vi "Save Properties as XML.vi"(8 "error in":errorcluster, 9 "Methods[]":T1(array[cluster]), 10 "Properties[]":T2(array[cluster]), 11 "Classes":T3(array[cluster])) -> (0 "error out":errorcluster)   [LabVIEW 2023]
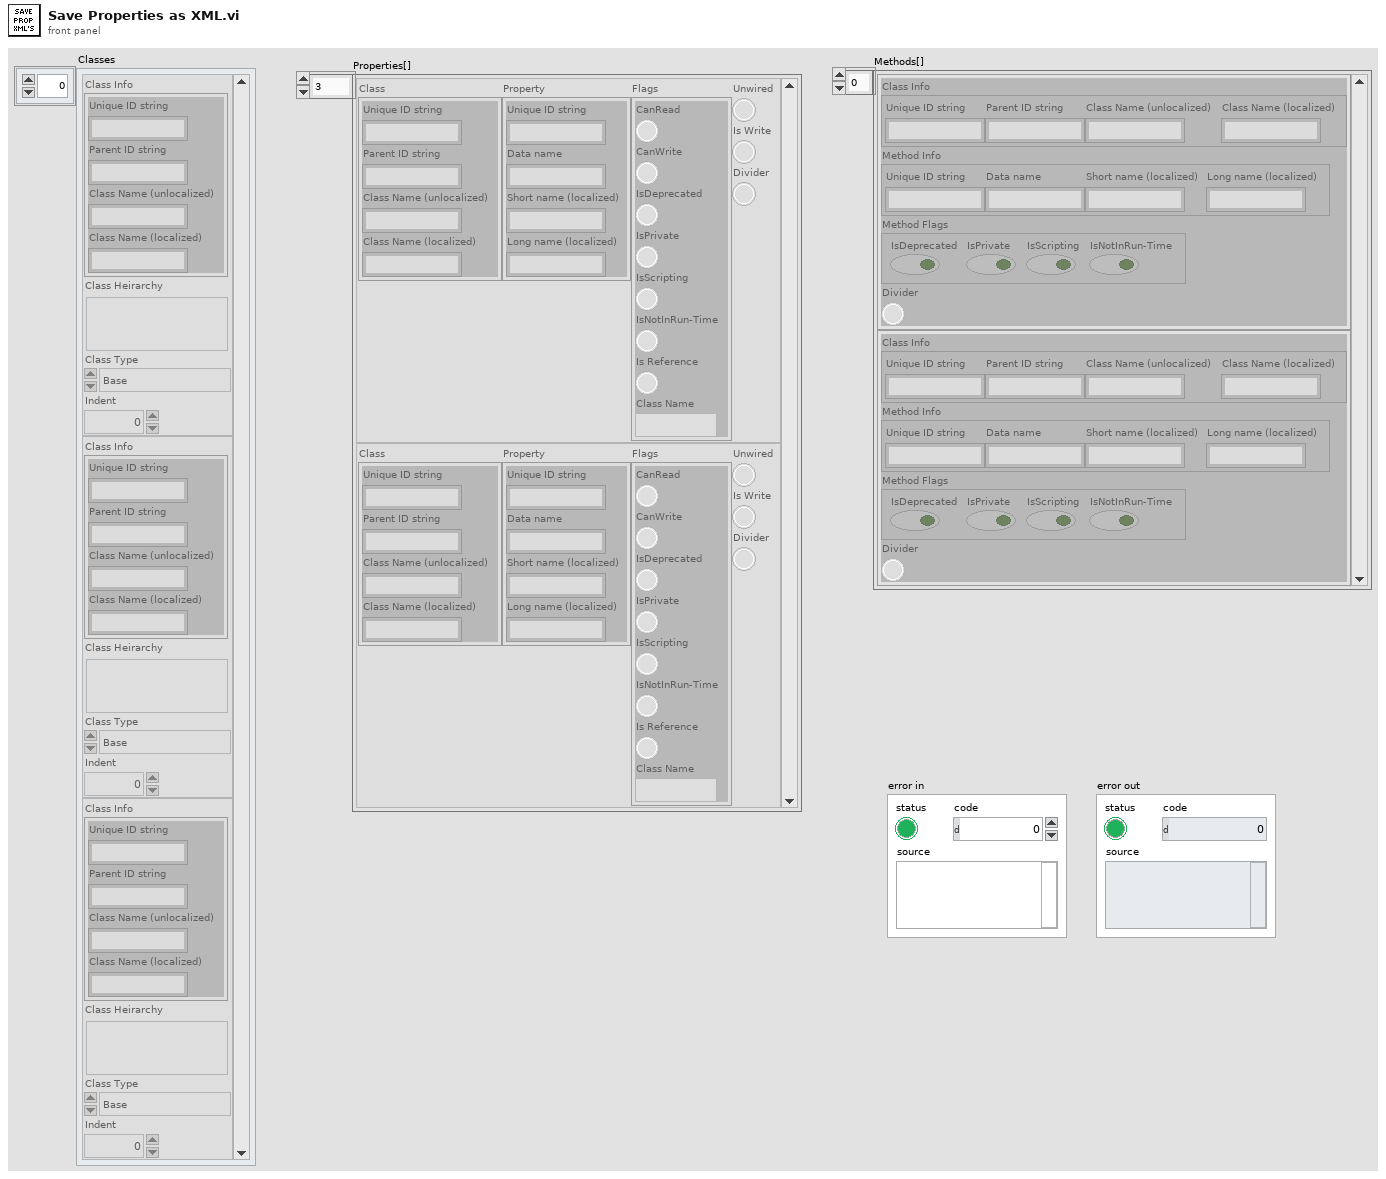
[diagram p1: front panel]
types:
  T1 = cluster{"Class Info":cluster{"Unique ID string":string, "Parent ID string":string, "Class Name (unlocalized)":string, "Class Name (localized)":string}, "Method Info":cluster{"Unique ID string":string, "Data name":string, "Short name (localized)":string, "Long name (localized)":string}, "Method Flags":cluster{"IsDeprecated":bool, "IsPrivate":bool, "IsScripting":bool, "IsNotInRun-Time":bool}, "Divider":bool}[]
  T2 = cluster{"Class":cluster{"Unique ID string":string, "Parent ID string":string, "Class Name (unlocalized)":string, "Class Name (localized)":string}, "Property":cluster{"Unique ID string":string, "Data name":string, "Short name (localized)":string, "Long name (localized)":string}, "Flags":cluster{"CanRead":bool, "CanWrite":bool, "IsDeprecated":bool, "IsPrivate":bool, "IsScripting":bool, "IsNotInRun-Time":bool, "Is Reference":bool, "Class Name":string}, "Divider":bool, "Is Write":bool, "Unwired":bool}[]
  T3 = cluster{"Class Info":cluster{"Unique ID string":string, "Parent ID string":string, "Class Name (unlocalized)":string, "Class Name (localized)":string}, "Class Heirarchy":string, "Class Type":enum16{"Unknown", "Base", "Scripting", "Private", "Deprecated", "None", "Divider"}, "Indent":u32}[]
  T4 = enum16{"open", "replace", "create", "open or create", "replace or create", "replace or create with confirmation"}
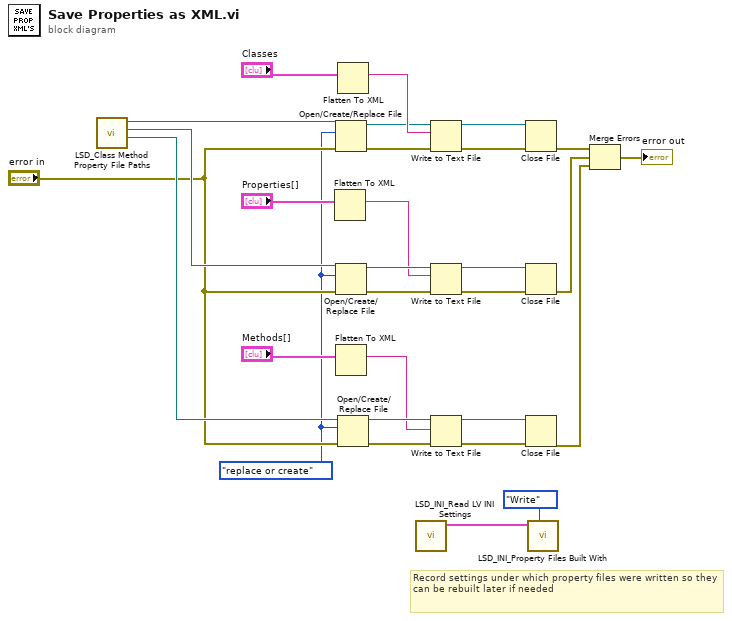
[diagram p0: block diagram]
diagram:
  w3 = T4."replace or create" ("operation (0:open)")
  # "Record settings under which property files were written so they can be rebuilt later if needed"
  n1 = call <resource>:"LSD_Class Method Property File Paths.vi"() -> ("Method Ini"=w5:path, "Property Ini"=w6:path, "Class Ini"=w7:path)  [unwired: 7 in, 2 out]
  n2 = Flatten To XML(6:"Properties[]") -> (2:w9:string)
  n3 = Open/Create/Replace File(file path (use dialog)=w7, error in="error in", operation (0:open)=w3) -> (refnum out=w22:refnum<file>, error out=w25:errorcluster)  [unwired: 3 in, 1 out]
  n4 = Open/Create/Replace File(file path (use dialog)=w6, error in="error in", operation (0:open)=w3) -> (refnum out=w17:refnum<file>, error out=w16:errorcluster)  [unwired: 3 in, 1 out]
  n5 = Flatten To XML(6:"Methods[]") -> (2:w8:string)
  n6 = Flatten To XML(6:"Classes") -> (2:w23:string)
  n7 = Open/Create/Replace File(file path (use dialog)=w5, error in="error in", operation (0:open)=w3) -> (refnum out=w13:refnum<file>, error out=w12:errorcluster)  [unwired: 3 in, 1 out]
  n8 = call <resource>:"LSD_INI_Read LV INI Settings.vi"() -> ("LabVIEW INI Settings"=w2:cluster{"Scripting":bool, "Private":bool})  [unwired: 10 in, 1 out]
  n9 = Write to Text File(file (use dialog)=w22, text=w23, error in=w25) -> (refnum out=w21:refnum<file>, error out=w24:errorcluster)  [unwired: 1 in, 1 out]
  n10 = Write to Text File(file (use dialog)=w17, text=w9, error in=w16) -> (refnum out=w15:refnum<file>, error out=w14:errorcluster)  [unwired: 1 in, 1 out]
  n11 = Write to Text File(file (use dialog)=w13, text=w8, error in=w12) -> (refnum out=w11:refnum<file>, error out=w10:errorcluster)  [unwired: 1 in, 1 out]
  n12 = Close File(refnum=w21, error in=w24) -> (error out=w29:errorcluster)  [unwired: 1 out]
  n13 = Close File(refnum=w15, error in=w14) -> (error out=w28:errorcluster)  [unwired: 1 out]
  n14 = Close File(refnum=w11, error in=w10) -> (error out=w27:errorcluster)  [unwired: 1 out]
  n15 = call <resource>:"LSD_INI_Property Files Built With.vi"("File Action"=enum16{"Read", "Write"}."Write", "Property Files Built With"=w2) -> ()  [unwired: 9 in, 1 out]
  n16 = Merge Errors(w29, w28, w27) -> (→"error out":errorcluster)
